vi "Actor Core.vi"(8 "error in":errorcluster, 11 "Main in":refnum<class "Main.lvclass">) -> (0 "error out":errorcluster, 3 "Actor out":refnum<class "Actor.lvclass">)   [LabVIEW 2023, in "GUI.lvlib" / "Main.lvlib" / "Main.lvclass"]
doc: "(<B>Filename</B>: Actor Framework.lvlib:Actor.lvclass:Actor Core.vi)\n\nReceives messages to the actor, reacts to them, and initiates any error handling that may shut the actor down.\n\nDescendant classes may override this VI to append parallel tasks for the actor to complete while it handles messages. Overrides use the Call Parent Method node."
uses:
  Main.lvclass
  <vilib>/ActorFramework/Actor/Actor.lvclass
  HardwareAbstractionLayer_LVOOP/Database/SQL Public VI/Control/DB Options.ctl
  Typdefs/Main.App.Cluster.ctl
  Main.lvclass/Main.ctl
  <vilib>/ActorFramework/Actor/Actor.lvclass/Actor.ctl
  <vilib>/ActorFramework/Message Enqueuer/Message Enqueuer.lvclass/Message Enqueuer.ctl
  Main Messages/Launch Nested Actors Selector Msg/Launch Nested Actors Selector Msg.lvclass/Launch Nested Actors Selector Msg.ctl
  <vilib>/ActorFramework/Message Enqueuer/Init from Existing Queue.vi
  <vilib>/ActorFramework/Message Enqueuer/Enqueue.vi
  Main Messages/Initialize Msg/Initialize Msg.lvclass
  Main Messages/Login and Logout Msg/Login and Logout Msg.lvclass
  Main Messages/Close panel Msg/Close panel Msg.lvclass
  Main Messages/Launch Nested Actors Selector Msg/Launch Nested Actors Selector Msg.lvclass
  <vilib>/ActorFramework/Message Priority Queue/Priority Enqueue.vi
  <vilib>/ActorFramework/Message Enqueuer/Message Enqueuer.lvclass
  GUI.lvlib
  HardwareAbstractionLayer_LVOOP/Error Handler/Error Handler_class/Error Handler.lvclass
  HardwareAbstractionLayer_LVOOP/Database/Database.lvclass
panel:
  in  "TestStand UI Application Manager":refnum<k7>(container)
  in  "Log in And Out":bool
  in  "Menubar":enum32{"Home", "Diagnostic", "Help", "Info"}(radio)
  in  "Stop":bool
  out "User":string="Coder "
  in  "Menu":bool
  out "Time":string="03:22:21 PM"
  out "Date":string="18/02/2019"
  in  "Close":bool
  out "User Level":string="Operator"
  out "Panel Name":string="Test Panel"
  in  "Sidebar":T1(radio)
  # "eDCU LIFE TIME TESTER"
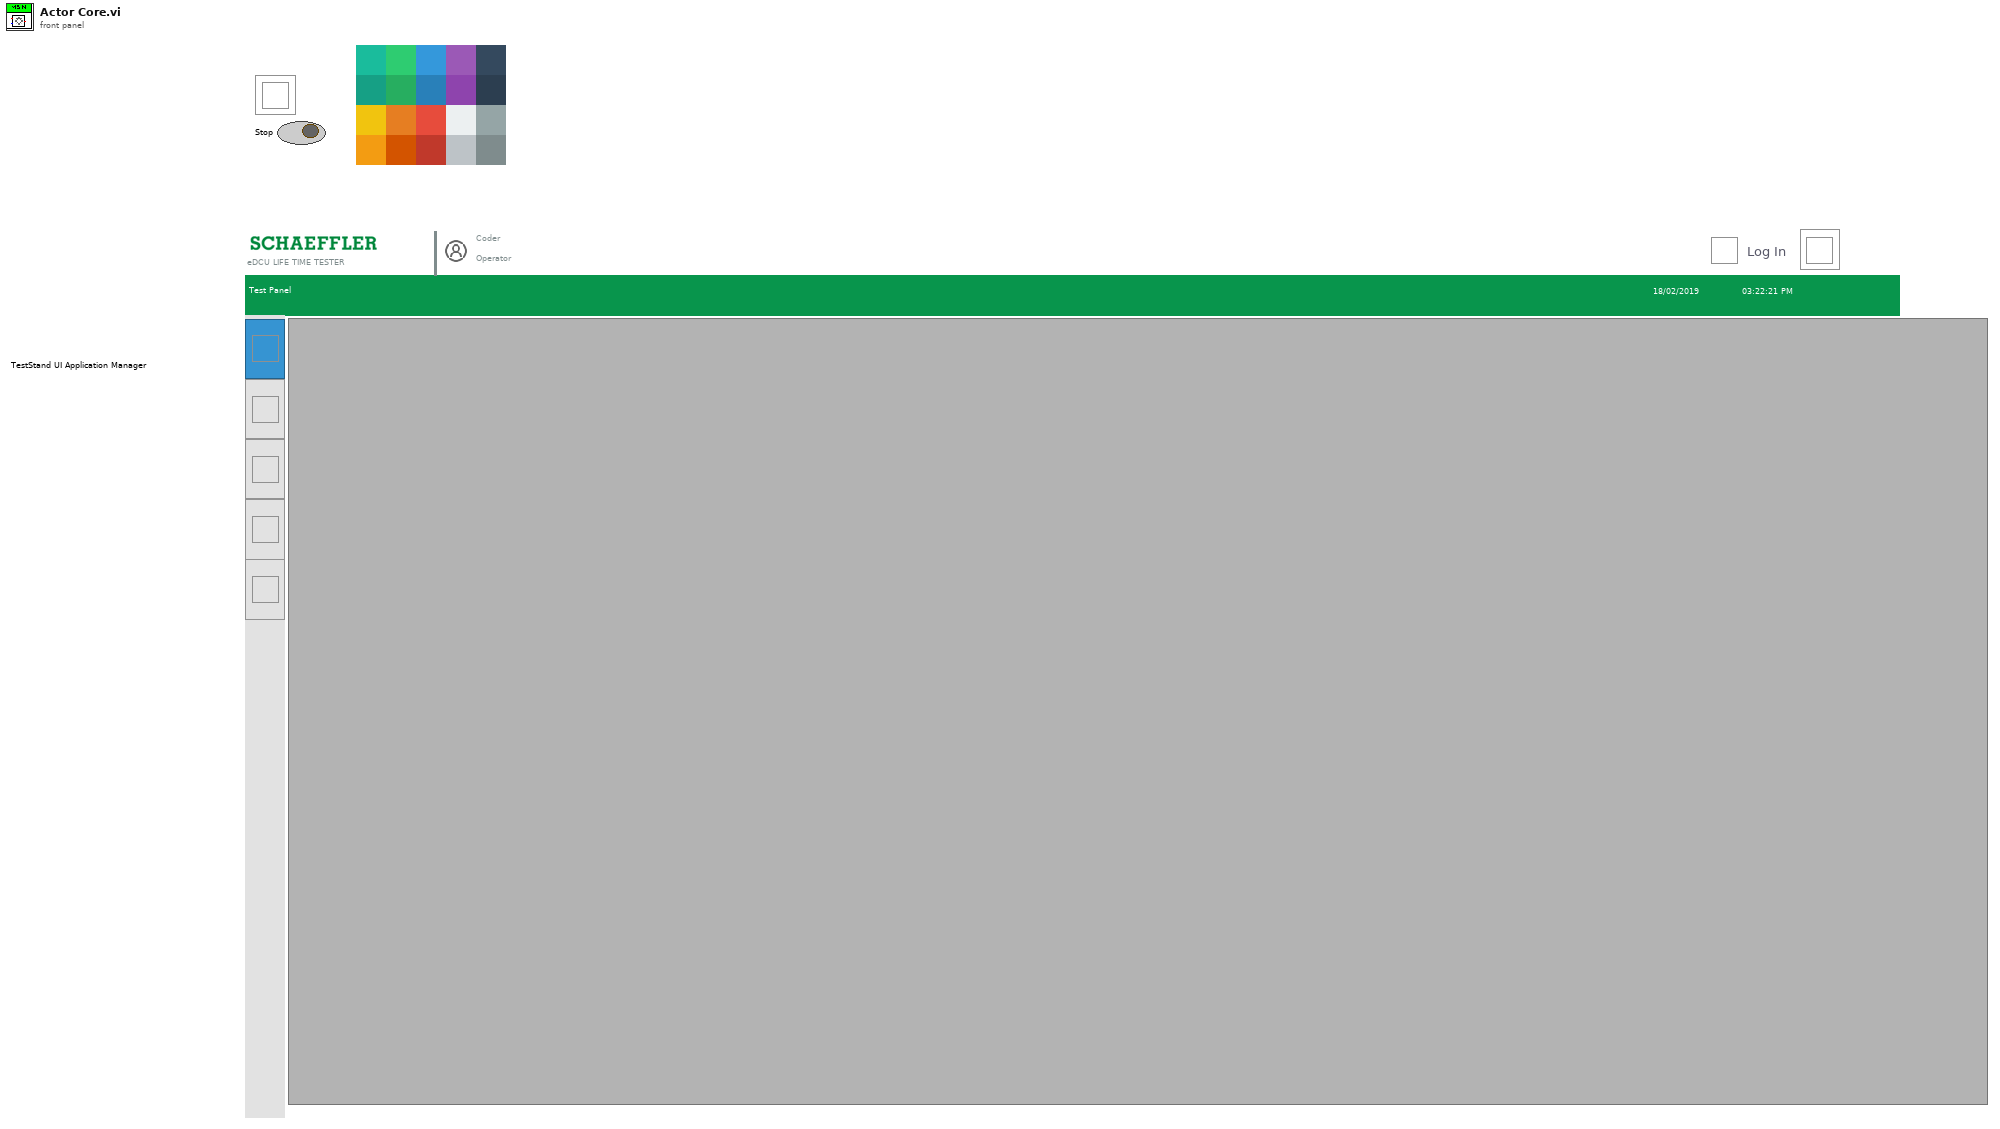
[diagram p1: front panel]
types:
  T1 = enum32{"Home", "Settings", "Diagnostic", "Help", "Info"}
  T2 = typedef "HardwareAbstractionLayer_LVOOP.lvlib/Database.lvclass/DB Options.ctl" = enum16{"Init", "Select Data", "Insert Data", "Update Data", "Delete Data", "Execute Query", "Create Schema", "Create Table", "List Tables", "List Columns", "Close"}
  T3 = typedef "GUI.lvlib/Main.App.Cluster.ctl" = cluster{"Sidebar":refnum<vi>, "Menubar":refnum<vi>, "Log in And Out":refnum<vi>, "User Level":refnum<vi>, "User":refnum<vi>, "Sub Panel":refnum<vi>, "Panel Name":refnum<vi>, "Menu":refnum<vi>, "Close":refnum<vi>}
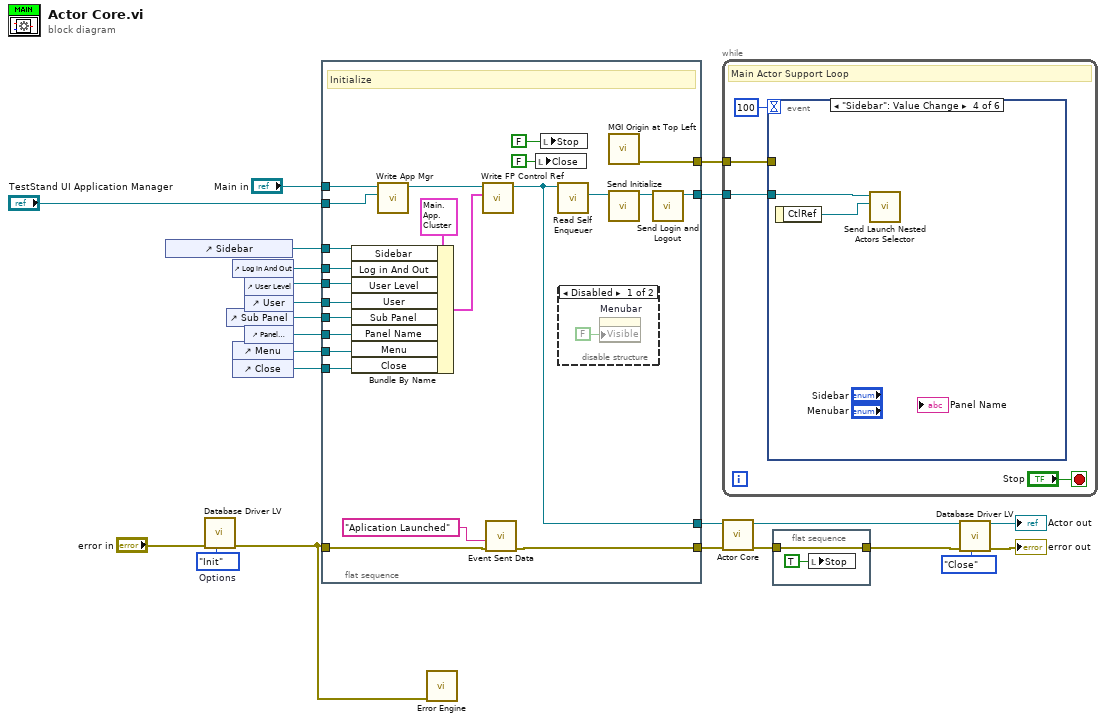
[diagram p0: block diagram]
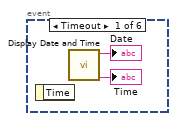
[diagram p3: hidden frame]
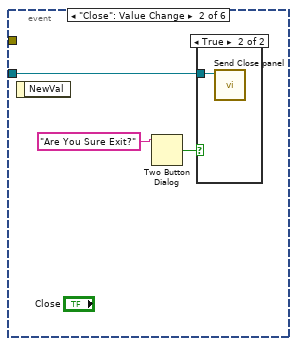
[diagram p4: hidden frame]
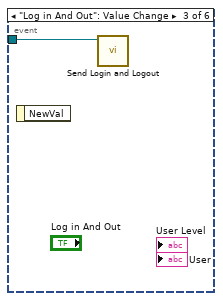
[diagram p6: hidden frame]
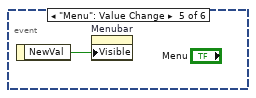
[diagram p7: hidden frame]
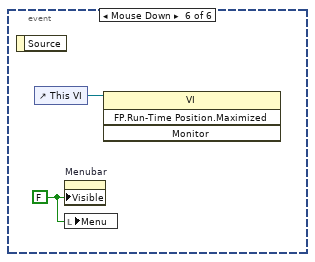
[diagram p8: hidden frame]
diagram:
  w1 = DB_Options."Init"  # Options
  n1 = control-ref of="Sidebar"() -> (w18:refnum<vi>)
  n2 = call "Database Driver LV.vi"("Options"=w1, "error in"="error in") -> ("error out"=w5:errorcluster)  [unwired: 6 in, 3 out]
  n3 = control-ref of="Sub Panel"() -> (w14:refnum<vi>)
  n4 = control-ref of="Log in And Out"() -> (w17:refnum<vi>)
  n5 = control-ref of="Menu"() -> (w12:refnum<vi>)
  n6 = control-ref of="Close"() -> (w11:refnum<vi>)
  n7 = control-ref of="User Level"() -> (w16:refnum<vi>)
  n8 = control-ref of="User"() -> (w15:refnum<vi>)
  n9 = control-ref of="Panel Name"() -> (w13:refnum<vi>)
  n10 = flat-sequence {
    tunnel: "Main in" -> [w31]
    tunnel: [w23] -> w20
    tunnel: [w44] -> w19
    tunnel: [w27] -> w8
    tunnel: w5 -> [w28]
    tunnel: [w45] -> w9
    tunnel: w18 -> [w42]
    tunnel: w17 -> [w41]
    tunnel: w16 -> [w40]
    tunnel: w15 -> [w39]
    tunnel: w14 -> [w38]
    tunnel: w13 -> [w37]
    tunnel: w12 -> [w36]
    tunnel: w11 -> [w32]
    tunnel: "TestStand UI Application Manager" -> [w25]
    frame #0 {
      # "Initialize"
      n11 = Bundle By Name(cluster=T3 {"Sidebar"=refnum, "Menubar"=refnum, "Log in And Out"=refnum, "User Level"=refnum, "User"=refnum, "Sub Panel"=refnum, "Panel Name"=refnum, "Menu"=refnum, "Close"=refnum} ("FP Control Ref"), "Sidebar"=w42, "Log in And Out"=w41, "User Level"=w40, "User"=w39, "Sub Panel"=w38, "Panel Name"=w37, "Menu"=w36, "Close"=w32) -> (w43:T3)
      n12 = call "Write App Mgr.vi"("App Mgr"=w25, "Main in"=w31) -> ("Main out"=w30:refnum<class "Main.lvclass">)  [unwired: 8 in, 1 out]
      n13 = call "Write FP Control Ref.vi"("FP Control Ref"=w43, "Main in"=w30) -> ("Main out"=w44:refnum<class "Main.lvclass">)  [unwired: 8 in, 1 out]
      n14 = call "Event Sent Data.vi"("error in"=w28, "EVENT Description"="Aplication Launched") -> ("error out"=w27:errorcluster)  [unwired: 9 in]
      n15 = local write "Close"(FALSE ("Close")) -> ()
      n16 = local write "Stop"(FALSE ("Stop")) -> ()
      n17 = call <vilib>:"Read Self Enqueuer.vi"("Actor"=w44) -> ("Self Enqueuer"=w33:refnum<class "Message Enqueuer.lvclass">)  [unwired: 10 in]
      n18 = disable-structure shown="Disabled" {
        frame Disabled {
          n19 = property on="Menubar" class="RadioBtnsControl (strict)"("Visible"=FALSE) -> ()  [unwired: 2 in, 2 out]
        }
        frame Enabled {
        }
      }
      n20 = call <userlib>:"MGI Origin at Top Left.vi"() -> ("Error Out"=w45:errorcluster)  [unwired: 9 in, 1 out]
      n21 = call "Send Initialize.vi"("Message Enqueuer"=w33) -> ("Message Enqueuer out"=w24:refnum<class "Message Enqueuer.lvclass">)  [unwired: 9 in, 1 out]
      n22 = call "Send Login and Logout.vi"("Message Enqueuer"=w24) -> ("Message Enqueuer out"=w23:refnum<class "Message Enqueuer.lvclass">)  [unwired: 9 in, 1 out]
    }
  }
  n23 = call "Error Engine.vi"("error in"=w5) -> ()  [unwired: 10 in, 1 out]
  n24 = while {
    tunnel: w20 -> [w48]
    tunnel: w9 -> [w47]
    stop <- "Stop" stop-if-true
    # "Main Actor Support Loop"
    n25 = event shown="[3] \"Sidebar\": Value Change" {
      selector: _ -> [_ _ _ _ _ _]
      dyn-events: _ -> [_ _ _ _ _ _]
      timeout: 100 -> [_ _ _ _ _ _]
      tunnel: w48 -> [_ w55 w57 w59 _ _]
      tunnel: w47 -> [_ _ _ _ _ _]
      event Timeout {
        n26 = event-data() -> ()  [unwired: 1 in, 1 out]
        n27 = call "Display Date and Time.vi"() -> ("Time"=→"Time":string, "Date"=→"Date":string)  [unwired: 10 in]
      }
      event "Close": Value Change {
        n28 = event-data() -> ()  [unwired: 1 in, 1 out]
        n29 = Two Button Dialog(message="Are You Sure Exit?") -> (T button?=w54:bool)  [unwired: 2 in]
        n30 = case shown="True" w54 {
          tunnel: w55 -> [_ w56]
          frame False {
          }
          frame True {
            n31 = call "Send Close panel.vi"("Message Enqueuer"=w56) -> ()  [unwired: 9 in, 2 out]
          }
        }
      }
      event "Log in And Out": Value Change {
        n32 = event-data() -> ()  [unwired: 1 in, 1 out]
        n33 = call "Send Login and Logout.vi"("Message Enqueuer"=w57) -> ()  [unwired: 9 in, 2 out]
      }
      event "Sidebar": Value Change {
        n34 = event-data() -> ("CtlRef"=w58:refnum<vi>)  [unwired: 1 in]
        n35 = call "Send Launch Nested Actors Selector.vi"("CTRL"=w58, "Message Enqueuer"=w59) -> ()  [unwired: 8 in, 2 out]
      }
      event "Menu": Value Change {
        n36 = event-data() -> ("NewVal"=w60:bool)  [unwired: 1 in]
        n37 = property on="Menubar" class="RadioBtnsControl (strict)"("Visible"=w60) -> ()  [unwired: 2 in, 2 out]
      }
      event Mouse Down {
        w62 = FALSE ("Visible")
        n38 = event-data() -> ()  [unwired: 1 in, 1 out]
        n39 = control-ref of="This VI"() -> (w61:refnum<vi>)
        n40 = property on="Menubar" class="RadioBtnsControl (strict)"("Visible"=w62) -> ()  [unwired: 2 in, 2 out]
        n41 = local write "Menu"(w62) -> ()
        n42 = invoke class="VI" method="FP.Run-Time Position.Maximized"(reference=w61) -> ()  [unwired: 3 in, 4 out]
      }
    }
  }
  n43 = call-parent "Actor Core.vi"("error in"=w8, "Actor in"=w19) -> ("error out"=w10:errorcluster, "Actor out"=→"Actor out":refnum<class "Actor.lvclass">)  [unwired: 8 in]
  n44 = flat-sequence {
    tunnel: w10 -> [w64]
    tunnel: [w64] -> w4
    frame #0 {
      n45 = local write "Stop"(TRUE ("Stop")) -> ()
    }
  }
  n46 = call "Database Driver LV.vi"("Options"=DB_Options."Close", "error in"=w4) -> ("error out"=→"error out":errorcluster)  [unwired: 6 in, 3 out]
